vi "sns scratchpad.vi"() -> ()   [LabVIEW 2015]
uses:
  Core/HTTP Request/Region.ctl
  Core/HTTP Request/AWS Credentials.ctl
  SMS/SMS Attribute Value Pair.ctl
  SMS/SMS Attribute.ctl
  SMS/SMS.lvclass
  Core/HTTP Request/HTTP Request.lvclass
panel:
  out "SMS Attributes":T1[](array[typedef])
  in  "AWS Credentials":T3
  in  "Region":T4
  out "error out":errorcluster
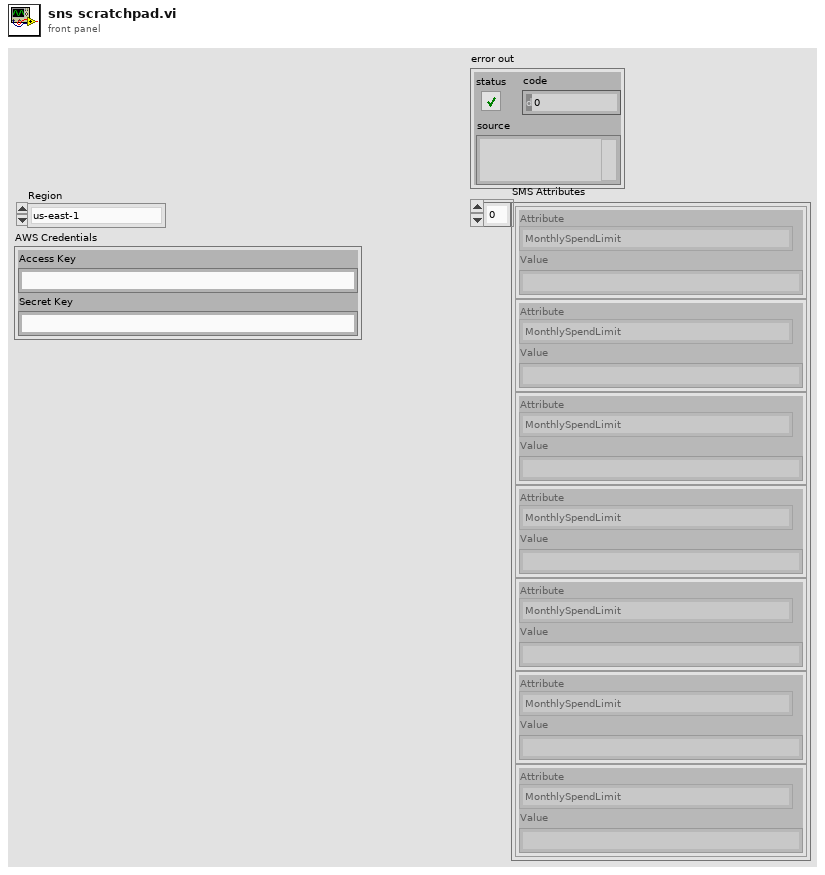
[diagram p1: front panel]
types:
  T1 = typedef "NI_AWS_SNS.lvlib/SMS.lvclass/SMS Attribute Value Pair.ctl" = cluster{"Attribute":T2, "Value":string}
  T2 = typedef "NI_AWS_SNS.lvlib/SMS.lvclass/SMS Attribute.ctl" = enum16{"MonthlySpendLimit", "DeliveryStatusIAMRole", "DeliveryStatusSuccessSamplingRate", "DefaultSenderID", "DefaultSMSType", "UsageReportS3Bucket"}
  T3 = typedef "NI_AWS_Core.lvlib/HTTP Request.lvclass/AWS Credentials.ctl" = cluster{"Access Key":string, "Secret Key":string}
  T4 = typedef "NI_AWS_Core.lvlib/HTTP Request.lvclass/Region.ctl" = enum16{"us-east-1", "us-east-2", "us-west-1", "us-west-2", "ap-northeast-1", "ap-northeast-2", "ap-southeast-1", "ap-southeast-2", "ca-central-1", "eu-central-1", "eu-west-1", "eu-west-2", "sa-east-1"}
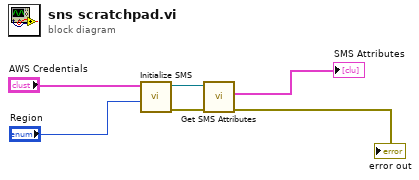
[diagram p0: block diagram]
diagram:
  n1 = call "Initialize SMS.vi"("Region"="Region", "AWS Credentials"="AWS Credentials") -> ("error out"=w3:errorcluster, "SMS"=w4:refnum<class "SMS.lvclass">)  [unwired: 8 in]
  n2 = call "Get SMS Attributes.vi"("error in (no error)"=w3, "SMS in"=w4) -> ("error out"=→"error out":errorcluster, "SMS Attributes"=→"SMS Attributes":T1[])  [unwired: 7 in, 1 out]
